vi "buffermgr.vi"(0 "Action":T2, 5 "buffer name":string, 7 "buffer size":u64, 9 "buffer pointer":u64, 11 "error in (no error)":errorcluster) -> (4 "output buffers":T1[](array[typedef]), 6 "output buffer":T1, 15 "error out":errorcluster)   [LabVIEW 2016]
uses:
  private/vis/BUFMGR_actionStruct.ctl
  private/vis/BufferStruct.ctl
panel:
  out "is locked?":bool
  in  "Buffers":T1[](array[typedef])
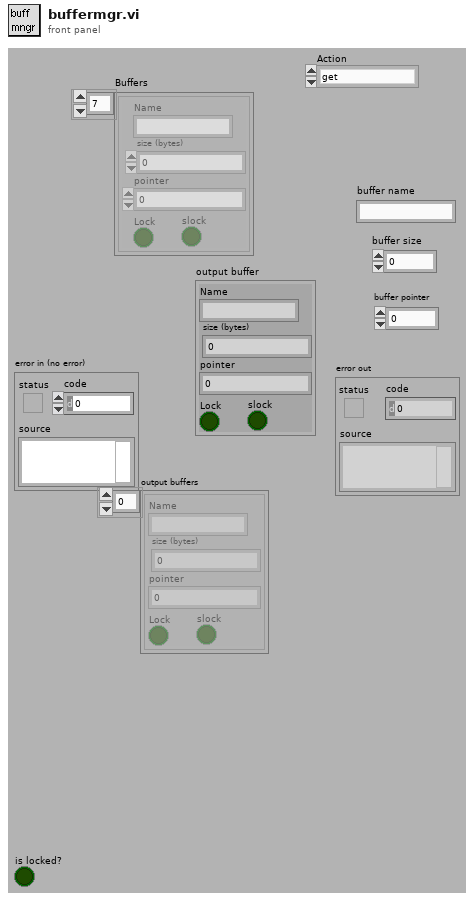
[diagram p1: front panel]
types:
  T1 = typedef "BufferStruct.ctl" = cluster{"Name":string, "size (bytes)":u64, "pointer":u64, "Lock":bool, "slock":bool}
  T2 = typedef "BUFMGR_actionStruct.ctl" = enum16{"get", "release", "get & lock", "unlock", "release all", "find", "release smaller than", "release bigger than", "release different than", "release equal to", "release unlocked", "info", "get & doublelock", "release secured", "double unlock"}
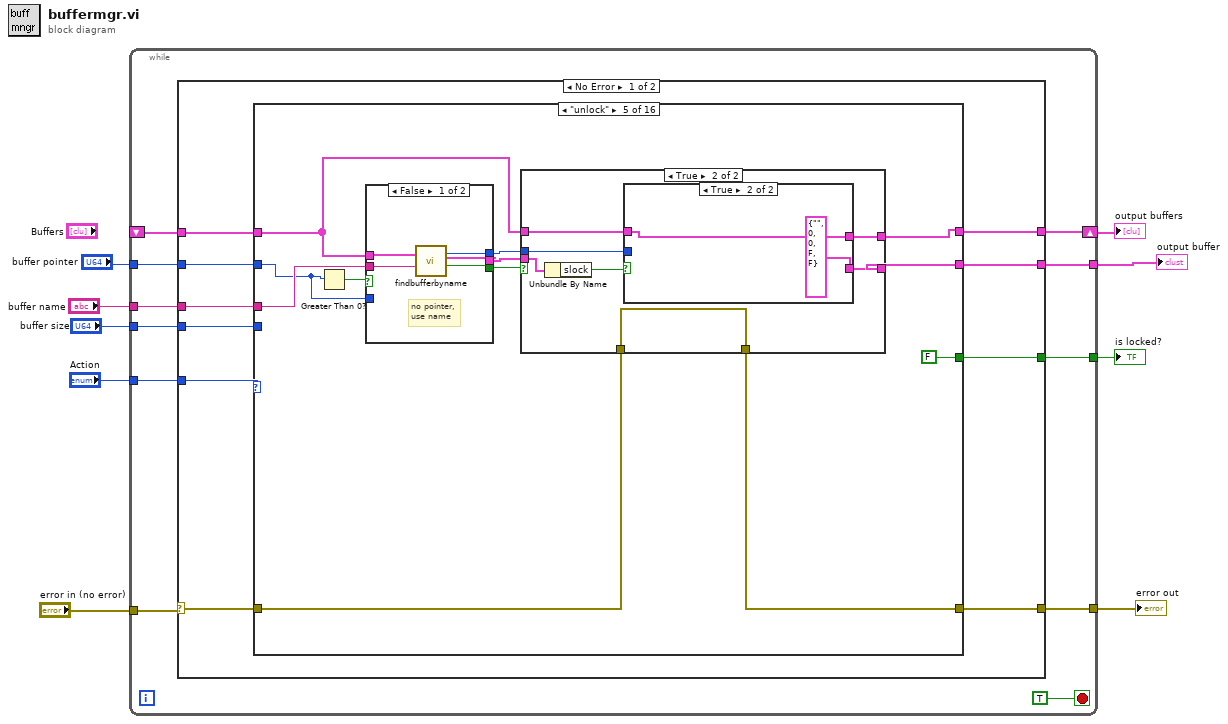
[diagram p0: block diagram]
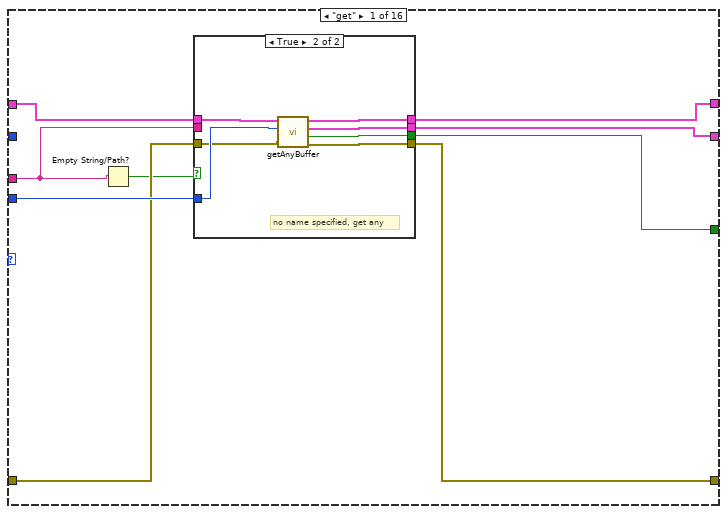
[diagram p2: hidden frame]
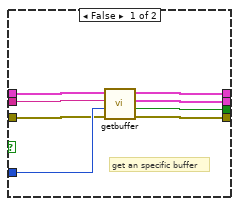
[diagram p3: hidden frame]
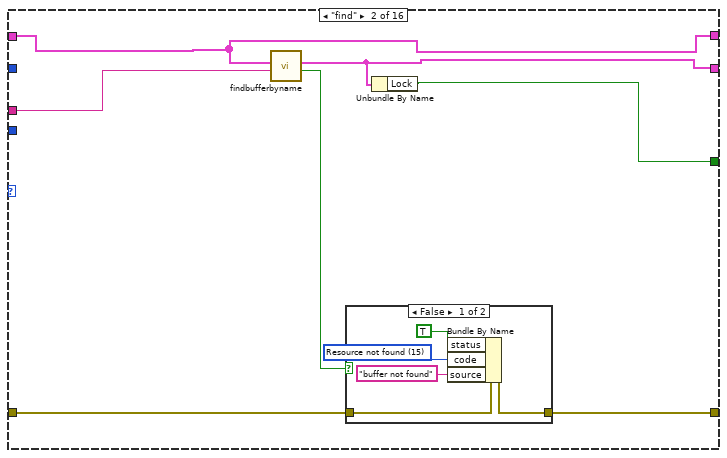
[diagram p4: hidden frame]
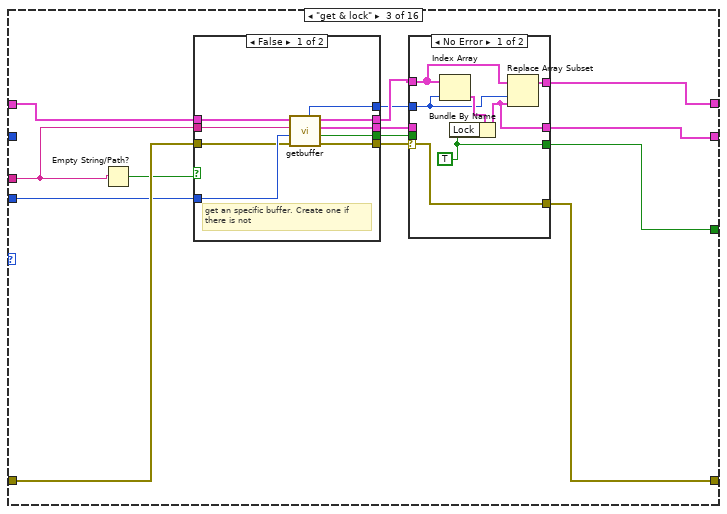
[diagram p6: hidden frame]
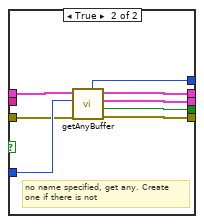
[diagram p8: hidden frame]
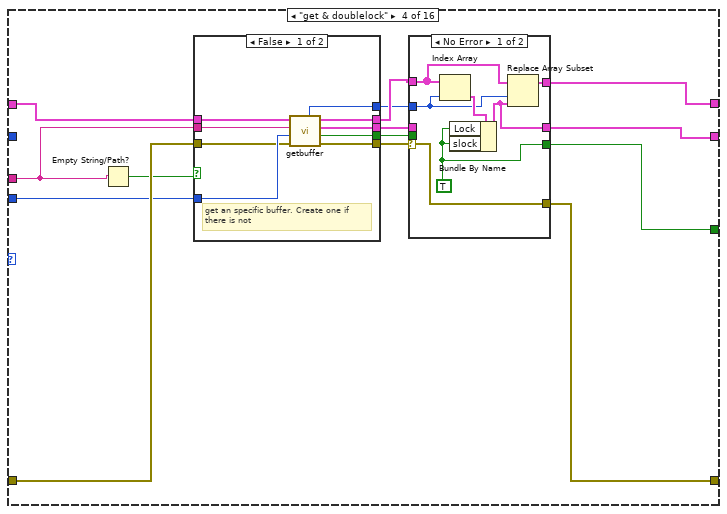
[diagram p9: hidden frame]
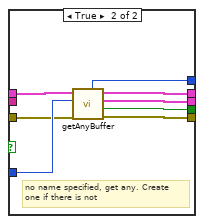
[diagram p11: hidden frame]
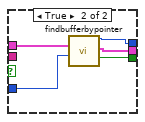
[diagram p12: hidden frame]
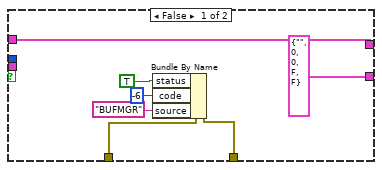
[diagram p13: hidden frame]
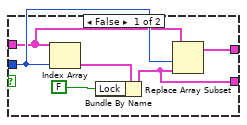
[diagram p14: hidden frame]
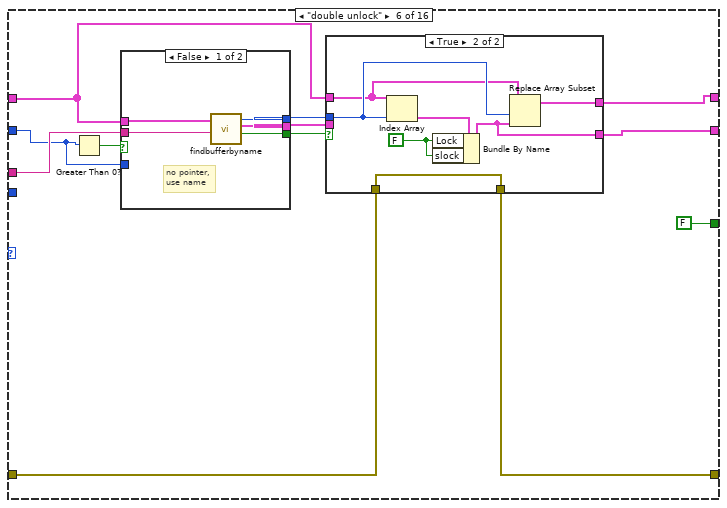
[diagram p15: hidden frame]
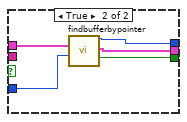
[diagram p16: hidden frame]
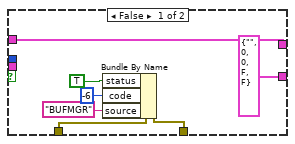
[diagram p17: hidden frame]
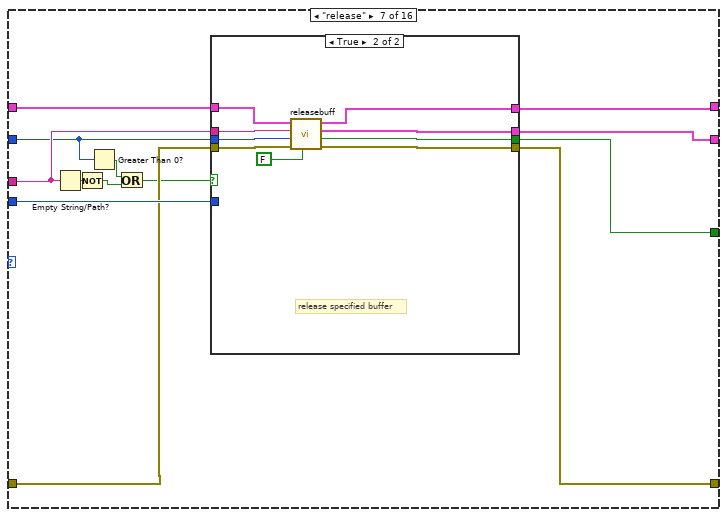
[diagram p18: hidden frame]
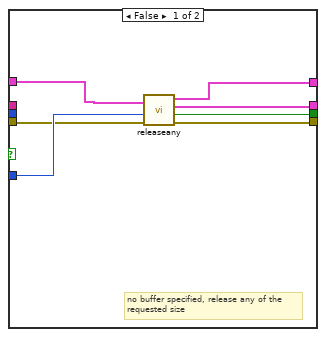
[diagram p19: hidden frame]
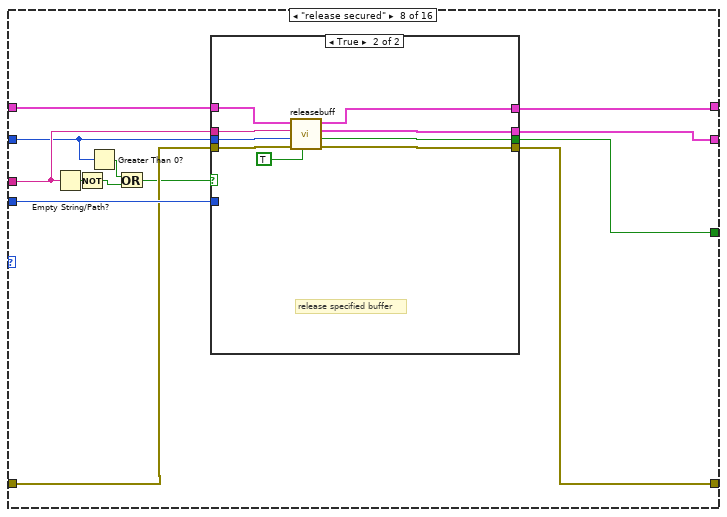
[diagram p20: hidden frame]
diagram:
  n1 = while {
    shift-left: _ -> [w11]
    shift-right: [w10] -> w2
    tunnel: "buffer pointer" -> [w13]
    tunnel: [w14] -> w4
    tunnel: [w15] -> w1
    tunnel: "buffer size" -> [w16]
    tunnel: "buffer name" -> [w17]
    tunnel: "Action" -> [w18]
    tunnel: [w19] -> w8
    tunnel: "error in (no error)" -> [w20]
    stop <- TRUE stop-if-true
    n2 = case shown="No Error" w20 {
      selector: w20 -> [w24 w466]
      tunnel: [w23 w466] -> w19
      tunnel: w11 -> [w21 w465]
      tunnel: w18 -> [w30 _]
      tunnel: w17 -> [w29 _]
      tunnel: w16 -> [w28 _]
      tunnel: [w27 w465] -> w10
      tunnel: [w26 T1 {"Name"="", "size (bytes)"=0, "pointer"=0, "Lock"=FALSE, "slock"=FALSE} ("output buffer")] -> w15
      tunnel: [w25 FALSE ("is locked")] -> w14
      tunnel: w13 -> [w22 _]
      frame No Error {
        n3 = case shown="\"unlock\"" w30 {
          tunnel: w21 -> [w38 w61 w81 w123 w157 w201 w243 w272 w296 w309 w343 w377 w411 w442 w456 w462]
          tunnel: w29 -> [w32 w60 w79 w121 w156 w200 w237 w266 _ w303 w337 w371 w405 _ _ _]
          tunnel: w28 -> [w39 _ w68 w110 _ _ w244 w273 _ w304 w338 w372 w406 _ _ _]
          tunnel: [w37 w61 w71 w113 w162 w206 w242 w271 w294 w307 w341 w375 w409 w440 w456 w462] -> w27
          tunnel: [w33 w59 w69 w111 w159 w203 w241 w270 T1 {"Name"="", "size (bytes)"=0, "pointer"=0, "Lock"=FALSE, "slock"=FALSE} ("output buffer") T1 {"Name"="", "size (bytes)"=0, "pointer"=0, "Lock"=FALSE, "slock"=FALSE} ("output buffer") T1 {"Name"="", "size (bytes)"=0, "pointer"=0, "Lock"=FALSE, "slock"=FALSE} ("output buffer") T1 {"Name"="", "size (bytes)"=0, "pointer"=0, "Lock"=FALSE, "slock"=FALSE} ("output buffer") T1 {"Name"="", "size (bytes)"=0, "pointer"=0, "Lock"=FALSE, "slock"=FALSE} ("output buffer") T1 {"Name"="", "size (bytes)"=0, "pointer"=0, "Lock"=FALSE, "slock"=FALSE} ("output buffer") T1 {"Name"="", "size (bytes)"=0, "pointer"=0, "Lock"=FALSE, "slock"=FALSE} ("output buffer") T1 {"Name"="", "size (bytes)"=0, "pointer"=0, "Lock"=FALSE, "slock"=FALSE} ("output buffer")] -> w26
          tunnel: [w34 w58 w70 w112 FALSE ("is locked") FALSE ("is locked") w238 w267 FALSE ("is locked") FALSE ("is locked") FALSE ("is locked") FALSE ("is locked") FALSE ("is locked") FALSE ("is locked") FALSE ("is locked") TRUE] -> w25
          tunnel: w24 -> [w36 w55 w80 w122 w153 w197 w240 w269 w292 w305 w339 w373 w407 w439 w457 w460]
          tunnel: [w35 w56 w76 w118 w152 w196 w239 w268 w292 w305 w339 w373 w407 w439 w457 w460] -> w23
          tunnel: w22 -> [_ _ _ _ w154 w198 w234 w263 _ _ _ _ _ _ _ _]
          frame "get" {
            n4 = Empty String/Path?(string/path=w32) -> (empty?=w31:bool)
            n5 = case shown="True" w31 {
              tunnel: w39 -> [w47 w53]
              tunnel: w38 -> [w46 w54]
              tunnel: [w45 w49] -> w37
              tunnel: w32 -> [w44 _]
              tunnel: w36 -> [w43 w52]
              tunnel: [w42 w48] -> w35
              tunnel: [w41 w51] -> w34
              tunnel: [w40 w50] -> w33
              frame False {
                # "get an specific buffer"
                n6 = call "getbuffer.vi"("error in"=w43, "buffer size"=w47, "buffer name"=w44, "Buffers"=w46) -> ("error out"=w42:errorcluster, "is locked"=w41:bool, "output buffer"=w40:T1, "Buffers out"=w45:T1[])  [unwired: 2 in, 2 out]
              }
              frame True {
                # "no name specified, get any"
                n7 = call "getAnyBuffer.vi"("error in"=w52, "buffer size"=w53, "Buffers"=w54) -> ("error out"=w48:errorcluster, "is locked"=w51:bool, "output buffer"=w50:T1, "output buffers"=w49:T1[])  [unwired: 5 out]
              }
            }
          }
          frame "find" {
            n8 = call "findbufferbyname.vi"("buffer name"=w60, "Buffers"=w61) -> ("found"=w57:bool, "buffer found"=w59:T1)  [unwired: 8 out]
            n9 = case shown="False" w57 {
              tunnel: w55 -> [w66 w67]
              tunnel: [w65 w67] -> w56
              frame False {
                w62 = 15 items=["No error", "Argument error", "Memory is full", "Out of zone", "End of file", "File already open", "Generic file I/O error", "File not found", "File permission error", "Disk is full", "Duplicate path", "Too many files open", "System feature not enabled", "Resource file not found", "Cannot add resource", "Resource not found", "Image not found", "Image memory error", "Pen does not exist", "Config type invalid", "Config token not found", "Config parse error", "Config memory error", "Bad external code format", "Bad external code offset", "External code not present", "Null window", "Destroy window error", "Null menu", "Print aborted", "Bad print record", "Print driver error", "Windows error during printing", "Memory error during printing", "Print dialog error", "Generic print error", "Invalid device refnum", "Device not found", "Device parameter error", "Device unit error", "Cannot open device", "Device call aborted", "Generic error", "Cancelled by user", "Object ID too low", "Object ID too high", "Object not in heap", "Unknown heap", "Unknown object (invalid DefProc)", "Unknown object (DefProc not in table)", "Message out of range", "Invalid (null) method", "Unknown message", "Manager call not supported", "Bad address", "Network operation in progress", "Network operation timed out", "Connection is busy", "Network attribute not supported", "Network error", "Address in use", "System out of memory", "Connection aborted", "Connection refused", "Not connected", "Already connected", "Connection closed", "Initialization error (interapplication manager)", "Bad occurrence", "Wait on unbound occurrence handler", "Occurrence queue overflow", "Datalog type conflict", "Unused", "Unrecognized type (interapplication manager)", "Memory corrupt", "Failed to make temporary DLL", "Old CIN version", "Drag socket not found", "Failed to load drop-object", "Failed to register OLE object", "Failed to release OLE object", "Format specifier type mismatch", "Unknown format specifier", "Too few format specifiers", "Too many format specifiers", "Scan failed", "Newer CIN version", "Error converting to variant", "Runtime menu error", "Password tampered", "Variant attribute not found", "Incompatible variant data type", "Event data is not available", "Event Store is not present", "Occurrence is not found", "Event Queue is not created", "Event info is not available", "Refnum passed is NULL", "Error retrieving Class GUID", "Error retrieving CoClass GUID", "Error retrieving TypeLib GUID.", "Bad built application magic bytes.", "Specific driver is different from the specific driver associated with the Logical Name.", "There is no session opened to the class driver.", "Max Error", "MAX - Error with config objects", "MAX - Error loading configuration", "MAX - Group not supported"]
                n10 = Bundle By Name(cluster=w66, "status"=TRUE, "code"=w62, "source"="buffer not found") -> (w65:errorcluster)
              }
              frame True {
              }
            }
            n11 = Unbundle By Name(w59) -> ("Lock"=w58:bool)
          }
          frame "get & lock" {
            n12 = Empty String/Path?(string/path=w79) -> (empty?=w78:bool)
            n13 = case shown="False" w78 {
              tunnel: w68 -> [w101 w108]
              tunnel: w81 -> [w100 w109]
              tunnel: [w99 w104] -> w75
              tunnel: w79 -> [w98 _]
              tunnel: w80 -> [w97 w107]
              tunnel: [w96 w103] -> w77
              tunnel: [w95 w106] -> w73
              tunnel: [w94 w105] -> w74
              tunnel: [w93 w102] -> w72
              frame False {
                # "get an specific buffer. Create one if \nthere is not"
                n14 = call "getbuffer.vi"("error in"=w97, "buffer size"=w101, "buffer name"=w98, "Buffers"=w100) -> ("error out"=w96:errorcluster, "is locked"=w95:bool, "output buffer"=w94:T1, "Buffers out"=w99:T1[], "index"=w93:i32)  [unwired: 2 in, 1 out]
              }
              frame True {
                # "no name specified, get any. Create\none if there is not"
                n15 = call "getAnyBuffer.vi"("error in"=w107, "buffer size"=w108, "Buffers"=w109) -> ("error out"=w103:errorcluster, "is locked"=w106:bool, "output buffer"=w105:T1, "output buffers"=w104:T1[], "index"=w102:i32)  [unwired: 4 out]
              }
            }
            n16 = case shown="No Error" w77 {
              selector: w77 -> [w86 w92]
              tunnel: [w86 w92] -> w76
              tunnel: w75 -> [w83 w91]
              tunnel: w74 -> [_ w89]
              tunnel: w73 -> [_ w90]
              tunnel: w72 -> [w82 _]
              tunnel: [w87 w91] -> w71
              tunnel: [w85 w90] -> w70
              tunnel: [w84 w89] -> w69
              frame No Error {
                w85 = TRUE ("Lock")
                n17 = Index Array(array=w83, index=w82) -> (element=w88:T1)
                n18 = Bundle By Name(cluster=w88, "Lock"=w85) -> (w84:T1)
                n19 = Replace Array Subset(array=w83, new element=w84, index=w82) -> (w87:T1[])
              }
              frame Error {
              }
            }
          }
          frame "get & doublelock" {
            n20 = Empty String/Path?(string/path=w121) -> (empty?=w120:bool)
            n21 = case shown="False" w120 {
              tunnel: w110 -> [w143 w150]
              tunnel: w123 -> [w142 w151]
              tunnel: [w141 w146] -> w117
              tunnel: w121 -> [w140 _]
              tunnel: w122 -> [w139 w149]
              tunnel: [w138 w145] -> w119
              tunnel: [w137 w148] -> w115
              tunnel: [w136 w147] -> w116
              tunnel: [w135 w144] -> w114
              frame False {
                # "get an specific buffer. Create one if \nthere is not"
                n22 = call "getbuffer.vi"("error in"=w139, "buffer size"=w143, "buffer name"=w140, "Buffers"=w142) -> ("error out"=w138:errorcluster, "is locked"=w137:bool, "output buffer"=w136:T1, "Buffers out"=w141:T1[], "index"=w135:i32)  [unwired: 2 in, 1 out]
              }
              frame True {
                # "no name specified, get any. Create\none if there is not"
                n23 = call "getAnyBuffer.vi"("error in"=w149, "buffer size"=w150, "Buffers"=w151) -> ("error out"=w145:errorcluster, "is locked"=w148:bool, "output buffer"=w147:T1, "output buffers"=w146:T1[], "index"=w144:i32)  [unwired: 4 out]
              }
            }
            n24 = case shown="No Error" w119 {
              selector: w119 -> [w128 w134]
              tunnel: [w128 w134] -> w118
              tunnel: w117 -> [w126 w133]
              tunnel: w116 -> [_ w131]
              tunnel: w115 -> [_ w132]
              tunnel: w114 -> [w125 _]
              tunnel: [w129 w133] -> w113
              tunnel: [w124 w132] -> w112
              tunnel: [w127 w131] -> w111
              frame No Error {
                w124 = TRUE ("Lock")
                n25 = Index Array(array=w126, index=w125) -> (element=w130:T1)
                n26 = Bundle By Name(cluster=w130, "Lock"=w124, "slock"=w124) -> (w127:T1)
                n27 = Replace Array Subset(array=w126, new element=w127, index=w125) -> (w129:T1[])
              }
              frame Error {
              }
            }
          }
          frame "unlock" {
            n28 = Greater Than 0?(x=w154) -> (x > 0?=w155:bool)
            n29 = case shown="False" w155 {
              tunnel: w156 -> [w168 _]
              tunnel: [w167 w171] -> w163
              tunnel: w157 -> [w166 w173]
              tunnel: [w165 w169] -> w161
              tunnel: [w164 w170] -> w158
              tunnel: w154 -> [_ w172]
              frame False {
                # "no pointer,\nuse name"
                n30 = call "findbufferbyname.vi"("buffer name"=w168, "Buffers"=w166) -> ("found"=w165:bool, "buffer found"=w164:T1, "index"=w167:i32)  [unwired: 7 out]
              }
              frame True {
                n31 = call "findbufferbypointer.vi"("pointer"=w172, "Buffers"=w173) -> ("found"=w169:bool, "buffer found"=w170:T1, "index"=w171:i32)  [unwired: 7 out]
              }
            }
            n32 = case shown="True" w161 {
              tunnel: w163 -> [_ w187]
              tunnel: w157 -> [w180 w186]
              tunnel: [w180 w185] -> w162
              tunnel: [T1 {"Name"="", "size (bytes)"=0, "pointer"=0, "Lock"=FALSE, "slock"=FALSE} ("buffer") w183] -> w159
              tunnel: w158 -> [_ w182]
              tunnel: w153 -> [w176 w184]
              tunnel: [w175 w184] -> w152
              frame False {
                n33 = Bundle By Name(cluster=w176, "status"=TRUE, "code"=-6, "source"="BUFMGR") -> (w175:errorcluster)
              }
              frame True {
                n34 = Unbundle By Name(w182) -> ("slock"=w181:bool)
                n35 = case shown="True" w181 {
                  tunnel: w187 -> [w191 _]
                  tunnel: w186 -> [w190 w195]
                  tunnel: [w189 w195] -> w185
                  tunnel: [w188 T1 {"Name"="", "size (bytes)"=0, "pointer"=0, "Lock"=FALSE, "slock"=FALSE} ("buffer")] -> w183
                  frame False {
                    n36 = Index Array(array=w190, index=w191) -> (element=w193:T1)
                    n37 = Bundle By Name(cluster=w193, "Lock"=FALSE) -> (w188:T1)
                    n38 = Replace Array Subset(array=w190, new element=w188, index=w191) -> (w189:T1[])
                  }
                  frame True {
                  }
                }
              }
            }
          }
          frame "double unlock" {
            n39 = Greater Than 0?(x=w198) -> (x > 0?=w199:bool)
            n40 = case shown="False" w199 {
              tunnel: w200 -> [w212 _]
              tunnel: [w211 w215] -> w207
              tunnel: w201 -> [w210 w217]
              tunnel: [w209 w213] -> w205
              tunnel: [w208 w214] -> w202
              tunnel: w198 -> [_ w216]
              frame False {
                # "no pointer,\nuse name"
                n41 = call "findbufferbyname.vi"("buffer name"=w212, "Buffers"=w210) -> ("found"=w209:bool, "buffer found"=w208:T1, "index"=w211:i32)  [unwired: 7 out]
              }
              frame True {
                n42 = call "findbufferbypointer.vi"("pointer"=w216, "Buffers"=w217) -> ("found"=w213:bool, "buffer found"=w214:T1, "index"=w215:i32)  [unwired: 7 out]
              }
            }
            n43 = case shown="True" w205 {
              tunnel: w207 -> [_ w230]
              tunnel: w201 -> [w224 w229]
              tunnel: [w224 w228] -> w206
              tunnel: [T1 {"Name"="", "size (bytes)"=0, "pointer"=0, "Lock"=FALSE, "slock"=FALSE} ("buffer") w226] -> w203
              tunnel: w202 -> [_ _]
              tunnel: w197 -> [w220 w227]
              tunnel: [w219 w227] -> w196
              frame False {
                n44 = Bundle By Name(cluster=w220, "status"=TRUE, "code"=-6, "source"="BUFMGR") -> (w219:errorcluster)
              }
              frame True {
                w225 = FALSE ("Lock")
                n45 = Index Array(array=w229, index=w230) -> (element=w231:T1)
                n46 = Bundle By Name(cluster=w231, "Lock"=w225, "slock"=w225) -> (w226:T1)
                n47 = Replace Array Subset(array=w229, new element=w226, index=w230) -> (w228:T1[])
              }
            }
          }
          frame "release" {
            n48 = Empty String/Path?(string/path=w237) -> (empty?=w236:bool)
            n49 = Not(x=w236) -> (.not. x?=w232:bool)
            n50 = Greater Than 0?(x=w234) -> (x > 0?=w233:bool)
            n51 = Or(x=w233, y=w232) -> (x .or. y?=w235:bool)
            n52 = case shown="True" w235 {
              tunnel: w244 -> [w249 _]
              tunnel: w243 -> [w251 w260]
              tunnel: [w250 w259] -> w242
              tunnel: [w245 w258] -> w241
              tunnel: w237 -> [_ w257]
              tunnel: w240 -> [w248 w256]
              tunnel: [w247 w255] -> w239
              tunnel: [w246 w254] -> w238
              tunnel: w234 -> [_ w253]
              frame False {
                # "no buffer specified, release any of the\nrequested size"
                n53 = call "releaseany.vi"("error in"=w248, "buffer size"=w249, "Buffers"=w251) -> ("error out"=w247:errorcluster, "is locked"=w246:bool, "output buffer"=w245:T1, "Buffers out"=w250:T1[])  [unwired: 3 in, 2 out]
              }
              frame True {
                # "release specified buffer"
                n54 = call "releasebuff.vi"("slock too?"=FALSE, "error in"=w256, "pointer"=w253, "buffer name"=w257, "Buffers"=w260) -> ("error out"=w255:errorcluster, "is locked"=w254:bool, "output buffer"=w258:T1, "Buffers out"=w259:T1[])  [unwired: 1 in, 2 out]
              }
            }
          }
          frame "release secured" {
            n55 = Empty String/Path?(string/path=w266) -> (empty?=w265:bool)
            n56 = Not(x=w265) -> (.not. x?=w261:bool)
            n57 = Greater Than 0?(x=w263) -> (x > 0?=w262:bool)
            n58 = Or(x=w262, y=w261) -> (x .or. y?=w264:bool)
            n59 = case shown="True" w264 {
              tunnel: w273 -> [w278 _]
              tunnel: w272 -> [w280 w289]
              tunnel: [w279 w288] -> w271
              tunnel: [w274 w287] -> w270
              tunnel: w266 -> [_ w286]
              tunnel: w269 -> [w277 w285]
              tunnel: [w276 w284] -> w268
              tunnel: [w275 w283] -> w267
              tunnel: w263 -> [_ w282]
              frame False {
                # "no buffer specified, release any of the\nrequested size"
                n60 = call "releaseany.vi"("error in"=w277, "buffer size"=w278, "Buffers"=w280) -> ("error out"=w276:errorcluster, "is locked"=w275:bool, "output buffer"=w274:T1, "Buffers out"=w279:T1[])  [unwired: 3 in, 2 out]
              }
              frame True {
                # "release specified buffer"
                n61 = call "releasebuff.vi"("slock too?"=TRUE, "error in"=w285, "pointer"=w282, "buffer name"=w286, "Buffers"=w289) -> ("error out"=w284:errorcluster, "is locked"=w283:bool, "output buffer"=w287:T1, "Buffers out"=w288:T1[])  [unwired: 1 in, 2 out]
              }
            }
          }
          frame "release all" {
            n62 = call "toFramemgr.vi"("command"="deleteall", "error in"=w292) -> ("error out"=w291:errorcluster)  [unwired: 7 in, 6 out]
            n63 = for {
              tunnel: w296 -> [w301] mode=indexing
              shift-right: [w298] -> w294
              shift-left: w296 -> [w299]
              tunnel: w291 -> [_]
              n64 = Unbundle By Name(w301) -> ("Name"=w300:string)
              n65 = call "releasebuff.vi"("slock too?"=TRUE, "buffer name"=w300, "Buffers"=w299) -> ("Buffers out"=w298:T1[])  [unwired: 3 in, 5 out]
            }
          }
          frame "release smaller than" {
            n66 = Greater Than 0?(x=w304) -> (x > 0?=w306:bool)
            n67 = case shown="True" w306 {
              tunnel: w309 -> [w310 w316]
              tunnel: [w310 w315] -> w307
              tunnel: w304 -> [_ w314]
              tunnel: w303 -> [_ w313]
              frame False {
              }
              frame True {
                # "if no \"force\"argument is given, then it will not be released if it is locked.\n\"force\" overrides the lock condition"
                n68 = Equal?(x="force", y=w313) -> (x = y?=w311:bool)
                n69 = for {
                  tunnel: w316 -> [w327] mode=indexing
                  shift-right: [w328] -> w315
                  shift-left: w316 -> [w329]
                  tunnel: w314 -> [w326]
                  tunnel: w311 -> [w321]
                  n70 = Unbundle By Name(w327) -> ("Name"=w323:string, "pointer"=w324:u64, "size (bytes)"=w325:u64, "Lock"=w322:bool)
                  n71 = Not(x=w322) -> (.not. x?=w319:bool)
                  n72 = Less?(x=w325, y=w326) -> (x < y?=w318:bool)
                  n73 = Select(t=w321, s=w321, f=w319) -> (s? t:f=w320:bool)
                  n74 = And(x=w318, y=w320) -> (x .and. y?=w317:bool)
                  n75 = case shown="True" w317 {
                    tunnel: w329 -> [w330 w335]
                    tunnel: [w330 w334] -> w328
                    tunnel: w324 -> [_ w333]
                    tunnel: w323 -> [_ w332]
                    frame False {
                    }
                    frame True {
                      n76 = call "releasebuff.vi"("slock too?"=FALSE, "pointer"=w333, "buffer name"=w332, "Buffers"=w335) -> ("Buffers out"=w334:T1[])  [unwired: 2 in, 5 out]
                    }
                  }
                }
              }
            }
          }
          frame "release bigger than" {
            n77 = Greater Than 0?(x=w338) -> (x > 0?=w340:bool)
            n78 = case shown="True" w340 {
              tunnel: w343 -> [w344 w350]
              tunnel: [w344 w349] -> w341
              tunnel: w338 -> [_ w348]
              tunnel: w337 -> [_ w347]
              frame False {
              }
              frame True {
                # "if no \"force\"argument is given, then it will not be released if it is locked.\n\"force\" overrides the lock condition"
                n79 = Equal?(x="force", y=w347) -> (x = y?=w345:bool)
                n80 = for {
                  tunnel: w350 -> [w361] mode=indexing
                  shift-right: [w362] -> w349
                  shift-left: w350 -> [w363]
                  tunnel: w348 -> [w360]
                  tunnel: w345 -> [w355]
                  n81 = Unbundle By Name(w361) -> ("Name"=w357:string, "pointer"=w358:u64, "size (bytes)"=w359:u64, "Lock"=w356:bool)
                  n82 = Not(x=w356) -> (.not. x?=w353:bool)
                  n83 = Greater?(x=w359, y=w360) -> (0:w352:bool)
                  n84 = Select(t=w355, s=w355, f=w353) -> (s? t:f=w354:bool)
                  n85 = And(x=w352, y=w354) -> (x .and. y?=w351:bool)
                  n86 = case shown="True" w351 {
                    tunnel: w363 -> [w364 w369]
                    tunnel: [w364 w368] -> w362
                    tunnel: w358 -> [_ w367]
                    tunnel: w357 -> [_ w366]
                    frame False {
                    }
                    frame True {
                      n87 = call "releasebuff.vi"("slock too?"=FALSE, "pointer"=w367, "buffer name"=w366, "Buffers"=w369) -> ("Buffers out"=w368:T1[])  [unwired: 2 in, 5 out]
                    }
                  }
                }
              }
            }
          }
          frame "release different than" {
            n88 = Greater Than 0?(x=w372) -> (x > 0?=w374:bool)
            n89 = case shown="True" w374 {
              tunnel: w377 -> [w378 w384]
              tunnel: [w378 w383] -> w375
              tunnel: w372 -> [_ w382]
              tunnel: w371 -> [_ w381]
              frame False {
              }
              frame True {
                # "if no \"force\"argument is given, then it will not be released if it is locked.\n\"force\" overrides the lock condition"
                n90 = Equal?(x="force", y=w381) -> (x = y?=w379:bool)
                n91 = for {
                  tunnel: w384 -> [w395] mode=indexing
                  shift-right: [w396] -> w383
                  shift-left: w384 -> [w397]
                  tunnel: w382 -> [w394]
                  tunnel: w379 -> [w389]
                  n92 = Unbundle By Name(w395) -> ("Name"=w391:string, "pointer"=w392:u64, "size (bytes)"=w393:u64, "Lock"=w390:bool)
                  n93 = Not(x=w390) -> (.not. x?=w387:bool)
                  n94 = Not Equal?(x=w393, y=w394) -> (x != y?=w386:bool)
                  n95 = Select(t=w389, s=w389, f=w387) -> (s? t:f=w388:bool)
                  n96 = And(x=w386, y=w388) -> (x .and. y?=w385:bool)
                  n97 = case shown="True" w385 {
                    tunnel: w397 -> [w398 w403]
                    tunnel: [w398 w402] -> w396
                    tunnel: w392 -> [_ w401]
                    tunnel: w391 -> [_ w400]
                    frame False {
                    }
                    frame True {
                      n98 = call "releasebuff.vi"("slock too?"=FALSE, "pointer"=w401, "buffer name"=w400, "Buffers"=w403) -> ("Buffers out"=w402:T1[])  [unwired: 2 in, 5 out]
                    }
                  }
                }
              }
            }
          }
          frame "release equal to" {
            n99 = Greater Than 0?(x=w406) -> (x > 0?=w408:bool)
            n100 = case shown="True" w408 {
              tunnel: w411 -> [w412 w418]
              tunnel: [w412 w417] -> w409
              tunnel: w406 -> [_ w416]
              tunnel: w405 -> [_ w415]
              frame False {
              }
              frame True {
                # "if no \"force\"argument is given, then it will not be released if it is locked.\n\"force\" overrides the lock condition"
                n101 = Equal?(x="force", y=w415) -> (x = y?=w413:bool)
                n102 = for {
                  tunnel: w418 -> [w429] mode=indexing
                  shift-right: [w430] -> w417
                  shift-left: w418 -> [w431]
                  tunnel: w416 -> [w428]
                  tunnel: w413 -> [w423]
                  n103 = Unbundle By Name(w429) -> ("Name"=w425:string, "pointer"=w426:u64, "size (bytes)"=w427:u64, "Lock"=w424:bool)
                  n104 = Not(x=w424) -> (.not. x?=w421:bool)
                  n105 = Equal?(x=w427, y=w428) -> (x = y?=w420:bool)
                  n106 = Select(t=w423, s=w423, f=w421) -> (s? t:f=w422:bool)
                  n107 = And(x=w420, y=w422) -> (x .and. y?=w419:bool)
                  n108 = case shown="True" w419 {
                    tunnel: w431 -> [w432 w437]
                    tunnel: [w432 w436] -> w430
                    tunnel: w426 -> [_ w435]
                    tunnel: w425 -> [_ w434]
                    frame False {
                    }
                    frame True {
                      n109 = call "releasebuff.vi"("slock too?"=FALSE, "pointer"=w435, "buffer name"=w434, "Buffers"=w437) -> ("Buffers out"=w436:T1[])  [unwired: 2 in, 5 out]
                    }
                  }
                }
              }
            }
          }
          frame "release unlocked" {
            n110 = for {
              tunnel: w442 -> [w446] mode=indexing
              shift-right: [w447] -> w440
              shift-left: w442 -> [w448]
              n111 = Unbundle By Name(w446) -> ("Name"=w444:string, "pointer"=w445:u64, "Lock"=w443:bool)
              n112 = case shown="False" w443 {
                tunnel: w448 -> [w453 w454]
                tunnel: [w452 w454] -> w447
                tunnel: w445 -> [w451 _]
                tunnel: w444 -> [w450 _]
                frame False {
                  n113 = call "releasebuff.vi"("slock too?"=FALSE, "pointer"=w451, "buffer name"=w450, "Buffers"=w453) -> ("Buffers out"=w452:T1[])  [unwired: 2 in, 5 out]
                }
                frame True {
                }
              }
            }
          }
          frame "info" {
          }
          frame Default {
          }
        }
      }
      frame Error {
      }
    }
  }
  "error out" <- w8
  "output buffers" <- w2
  "output buffer" <- w1
  "is locked?" <- w4
